vi "tt20panel_DO_stream_data.vi"(7 "Overwrite?":bool, 8 "error in (no error)":errorcluster, 9 "stream_settings":T1, 10 "stop_counts":refnum<queue>, 11 "tt20panel in":refnum<class "tt20panel.lvclass">) -> (0 "error out":errorcluster, 3 "tt20panel out":refnum<class "tt20panel.lvclass">)   [LabVIEW 2015, in "tt20panel.lvclass"]
uses:
  tt20panel.lvclass
  tt20_stream_settings_tdef.ctl
  tt20_class/tt20.lvclass
  tt20_logger_class/tt20_logger.lvclass
  Data Logger Class/data_logger.lvclass
  UI/panel_class/panel.lvclass
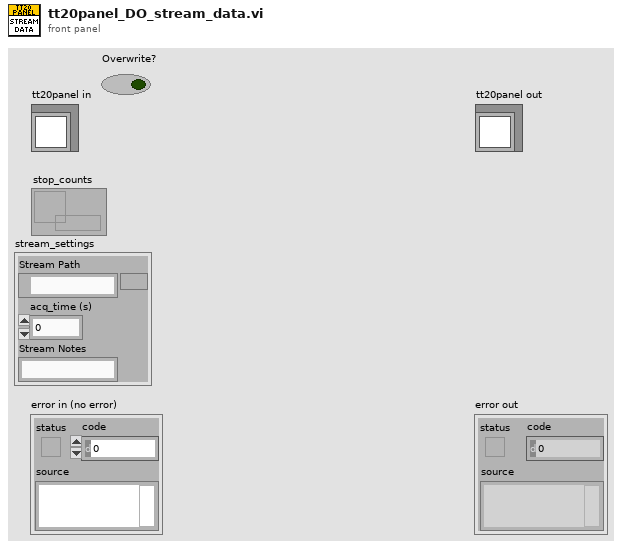
[diagram p1: front panel]
types:
  T1 = typedef "tt20_stream_settings_tdef.ctl" = cluster{"Stream Path":path, "acq_time (s)":u32, "Stream Notes":string}
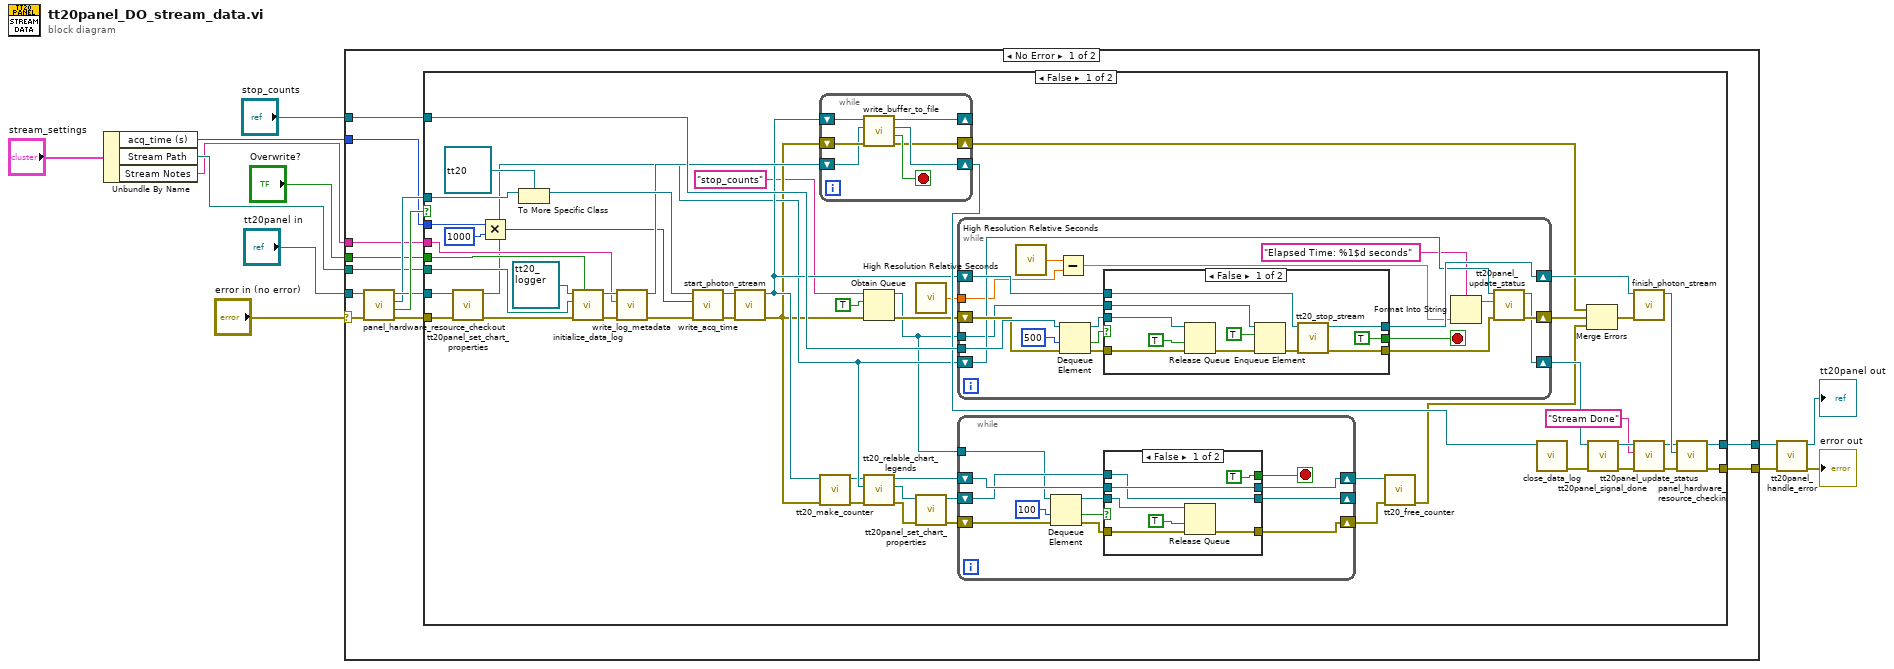
[diagram p0: block diagram]
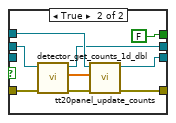
[diagram p2: hidden frame]
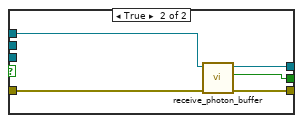
[diagram p3: hidden frame]
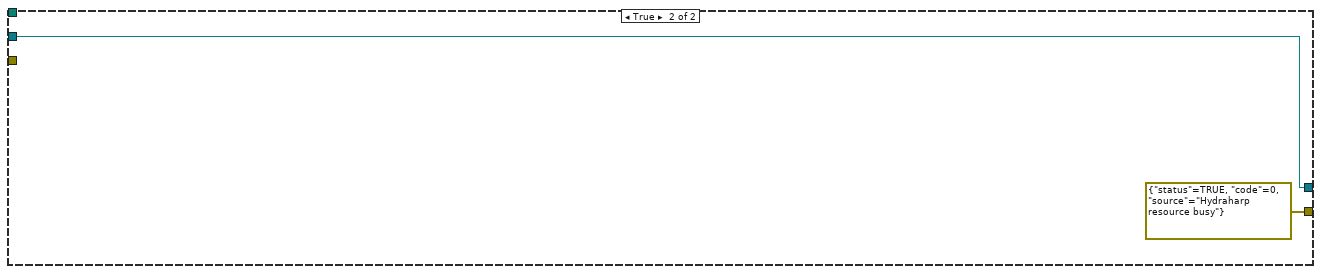
[diagram p4: hidden frame]
diagram:
  n1 = Unbundle By Name("stream_settings") -> ("acq_time (s)"=w4:u32, "Stream Path"=w3:path, "Stream Notes"=w1:string)
  n2 = case shown="No Error" "error in (no error)" {
    selector: "error in (no error)" -> [w24 w152]
    tunnel: [w21 w152] -> w10
    tunnel: [w18 w151] -> w6
    tunnel: "tt20panel in" -> [w25 w151]
    tunnel: "stop_counts" -> [w17 _]
    tunnel: w4 -> [w16 _]
    tunnel: w3 -> [w15 _]
    tunnel: "Overwrite?" -> [w14 _]
    tunnel: w1 -> [w13 _]
    frame No Error {
      n3 = call "panel_hardware_resource_checkout.vi"("error in (no error)"=w24, "panel in"=w25) -> ("error out"=w22:errorcluster, "timed out?"=w23:bool, "hardware.lvclass"=w19:refnum<class "hardware.lvclass">, "panel out"=w20:refnum<class "tt20panel.lvclass">)  [unwired: 6 in]
      n4 = case shown="False" w23 {
        tunnel: w22 -> [w75 _]
        tunnel: [w77 errorcluster {"status"=TRUE, "code"=0, "source"="Hydraharp resource busy"} ("error out")] -> w21
        tunnel: w20 -> [w74 w149]
        tunnel: w19 -> [w78 _]
        tunnel: [w76 w149] -> w18
        tunnel: w17 -> [w71 _]
        tunnel: w16 -> [w50 _]
        tunnel: w15 -> [w63 _]
        tunnel: w14 -> [w62 _]
        tunnel: w13 -> [w57 _]
        frame False {
          n5 = call "tt20panel_set_chart_properties.vi"("error in (no error)"=w75, "panel.lvclass"=w74) -> ("error in (no error) 2"=w65:errorcluster, "panel out"=w41:refnum<class "tt20panel.lvclass">)  [unwired: 8 in]
          n6 = Multiply(x=w50, y=u32 1000) -> (x*y=w48:u32)
          n7 = To More Specific Class(target class=refnum<class "tt20.lvclass"> refnum ("tt20.lvclass"), reference=w78) -> (specific class reference=w72:refnum<class "tt20.lvclass">)  [unwired: 1 in, 1 out]
          n8 = call-dynamic "initialize_data_log.vi"("Overwrite?"=w62, "error in (no error)"=w65, "Path"=w63, "tt20_logger in"=refnum<class "tt20_logger.lvclass"> refnum) -> ("error out"=w61:errorcluster, "tt20_logger out"=w59:refnum<class "tt20_logger.lvclass">)  [unwired: 6 in]
          n9 = call-dynamic "write_log_metadata.vi"("error in (no error)"=w61, "data"=w57, "tt20_logger in"=w59) -> ("error out"=w60:errorcluster, "tt20_logger out"=w58:refnum<class "tt20_logger.lvclass">)  [unwired: 7 in]
          n10 = call-dynamic "write_acq_time.vi"("error in (no error)"=w60, "acq_time_s"=w48, "tt20 in"=w72) -> ("error out"=w70:errorcluster, "tt20 out"=w73:refnum<class "tt20.lvclass">)  [unwired: 7 in]
          n11 = call-dynamic "start_photon_stream.vi"("error in (no error)"=w70, "tt20 in"=w73) -> ("error out"=w30:errorcluster, "tt20 out"=w42:refnum<class "tt20.lvclass">)  [unwired: 8 in]
          n12 = while {
            shift-right: [w111] -> _
            shift-left: w42 -> [w113]
            shift-right: [w107] -> w46
            shift-left: w30 -> [w110]
            shift-right: [w108] -> w68
            shift-left: w58 -> [w109]
            stop <- w112 stop-if-true
            n13 = call-dynamic "write_buffer_to_file.vi"("error in (no error)"=w110, "data_logger.lvclass"=w109, "tt20 in"=w113) -> ("error out"=w107:errorcluster, "Stream_done"=w112:bool, "data_logger.lvclass_out"=w108:refnum<class "data_logger.lvclass">, "tt20 out"=w111:refnum<class "tt20.lvclass">)  [unwired: 5 in]
          }
          n14 = call "tt20_make_counter.vi"("error in (no error)"=w30, "tt20 in"=w42) -> ("error out"=w37:errorcluster, "tt20 out"=w36:refnum<class "tt20.lvclass">)  [unwired: 8 in]
          n15 = Obtain Queue(name (unnamed)="stop_counts", element data type=TRUE, error in (no error)=w30) -> (queue out=w26:refnum<queue>, error out=w29:errorcluster)  [unwired: 2 in, 1 out]
          n16 = call "tt20_relable_chart_legends.vi"("error in (no error)"=w37, "panel in"=w41, "tt20 in"=w36) -> ("error out"=w33:errorcluster, "panel out"=w35:refnum<class "tt20panel.lvclass">, "tt20 out"=w34:refnum<class "tt20.lvclass">)  [unwired: 6 in]
          n17 = call <vilib>:"High Resolution Relative Seconds.vi"() -> ("relative seconds"=w43:dbl)
          n18 = call "tt20panel_set_chart_properties.vi"("error in (no error)"=w33, "panel.lvclass"=w35) -> ("error in (no error) 2"=w40:errorcluster, "panel out"=w39:refnum<class "tt20panel.lvclass">)  [unwired: 8 in]
          n19 = while {
            tunnel: w71 -> [w129]
            shift-right: [w131] -> w47
            shift-left: w42 -> [w132]
            shift-right: [w123] -> w45
            shift-left: w29 -> [w128]
            shift-right: [w121] -> w67
            shift-left: w41 -> [w122]
            tunnel: w43 -> [w117]
            tunnel: w26 -> [w114]
            stop <- w126 stop-if-true
            n20 = call <vilib>:"High Resolution Relative Seconds.vi"() -> ("relative seconds"=w116:dbl)
            n21 = Subtract(x=w116, y=w117) -> (x-y=w115:dbl)
            n22 = Dequeue Element(queue=w129, timeout in ms (-1)=500, error in (no error)=w128) -> (queue out=w125:refnum<queue>, timed out?=w127:bool, error out=w130:errorcluster)  [unwired: 1 out]
            n23 = case shown="False" w127 {
              tunnel: w132 -> [w138 w148]
              tunnel: [w137 w147] -> w131
              tunnel: w130 -> [w141 w146]
              tunnel: [TRUE w144] -> w126
              tunnel: [w139 w145] -> w124
              tunnel: w125 -> [w142 _]
              tunnel: w114 -> [w134 _]
              frame False {
                n24 = Release Queue(queue=w142, force destroy? (F)=TRUE, error in (no error)=w141) -> (error out=w136:errorcluster)  [unwired: 2 out]
                n25 = Enqueue Element(queue=w134, element=TRUE, error in (no error)=w136) -> (error out=w135:errorcluster)  [unwired: 1 in, 2 out]
                n26 = call "tt20_stop_stream.vi"("error in (no error)"=w135, "tt20 in"=w138) -> ("error out"=w139:errorcluster, "tt20 out"=w137:refnum<class "tt20.lvclass">)  [unwired: 8 in]
              }
              frame True {
                n27 = call-dynamic "receive_photon_buffer.vi"("error in (no error)"=w146, "tt20 in"=w148) -> ("error out"=w145:errorcluster, "done"=w144:bool, "tt20 out"=w147:refnum<class "tt20.lvclass">)  [unwired: 7 in]
              }
            }
            n28 = Format Into String(format string="Elapsed Time: %1$d seconds", w115) -> (resulting string=w118:string)  [unwired: 2 in, 1 out]
            n29 = call "tt20panel_update_status.vi"("error in (no error)"=w124, "status"=w118, "tt20panel in"=w122) -> ("error out"=w123:errorcluster, "tt20panel out"=w121:refnum<class "tt20panel.lvclass">)  [unwired: 7 in]
          }
          n30 = while {
            shift-right: [w83] -> w32
            shift-left: w40 -> [w89]
            shift-right: [w84] -> w38
            shift-left: w34 -> [w86]
            shift-right: [w82] -> _
            shift-left: w39 -> [w85]
            tunnel: w26 -> [w79]
            stop <- w81 stop-if-true
            n31 = Dequeue Element(queue=w79, timeout in ms (-1)=100, error in (no error)=w89) -> (queue out=w80:refnum<queue>, timed out?=w88:bool, error out=w87:errorcluster)  [unwired: 1 out]
            n32 = case shown="False" w88 {
              tunnel: w87 -> [w93 w106]
              tunnel: w86 -> [w96 w105]
              tunnel: w85 -> [w95 w104]
              tunnel: [w96 w101] -> w84
              tunnel: [w92 w100] -> w83
              tunnel: [w95 w99] -> w82
              tunnel: [TRUE FALSE] -> w81
              tunnel: w80 -> [w94 _]
              frame False {
                n33 = Release Queue(queue=w94, force destroy? (F)=TRUE, error in (no error)=w93) -> (error out=w92:errorcluster)  [unwired: 2 out]
              }
              frame True {
                n34 = call-dynamic "detector_get_counts_1d_dbl.vi"("error in (no error)"=w106, "tt20 in"=w105) -> ("error out"=w103:errorcluster, "counts"=w102:dbl[], "tt20 out"=w101:refnum<class "tt20.lvclass">)  [unwired: 7 in]
                n35 = call "tt20panel_update_counts.vi"("error in (no error)"=w103, "Counts"=w102, "tt20panel in"=w104) -> ("error out"=w100:errorcluster, "tt20panel out"=w99:refnum<class "tt20panel.lvclass">)  [unwired: 7 in]
              }
            }
          }
          n36 = call "tt20_free_counter.vi"("error in (no error)"=w32, "tt20 in"=w38) -> ("error out"=w31:errorcluster)  [unwired: 8 in, 1 out]
          n37 = call-dynamic "close_data_log.vi"("data_logger in"=w68) -> ("error out"=w69:errorcluster)  [unwired: 9 in, 1 out]
          n38 = Merge Errors(w46, w45, w31) -> (w44:errorcluster)
          n39 = call "tt20panel_signal_done.vi"("error in (no error)"=w69, "tt20panel in"=w67) -> ("error out"=w55:errorcluster, "tt20panel out"=w53:refnum<class "tt20panel.lvclass">)  [unwired: 8 in]
          n40 = call-dynamic "finish_photon_stream.vi"("error in (no error)"=w44, "tt20 in"=w47) -> ("tt20 out"=w56:refnum<class "tt20.lvclass">)  [unwired: 8 in, 1 out]
          n41 = call "tt20panel_update_status.vi"("error in (no error)"=w55, "status"="Stream Done", "tt20panel in"=w53) -> ("error out"=w54:errorcluster, "tt20panel out"=w52:refnum<class "tt20panel.lvclass">)  [unwired: 7 in]
          n42 = call "panel_hardware_resource_checkin.vi"("error in (no error)"=w54, "hardware.lvclass"=w56, "panel in"=w52) -> ("error out"=w77:errorcluster, "panel out"=w76:refnum<class "tt20panel.lvclass">)  [unwired: 7 in]
        }
        frame True {
        }
      }
    }
    frame Error {
    }
  }
  n43 = call "tt20panel_handle_error.vi"("error in (no error)"=w10, "tt20panel in"=w6) -> ("error out"=→"error out":errorcluster, "tt20panel out"=→"tt20panel out":refnum<class "tt20panel.lvclass">)  [unwired: 8 in]
